vi "QCA Get Message.vi"(0 "Timeout ms (-1)":i32=-1) -> (1 "QCA Message Type":T1(ring), 2 "Text":string)   [LabVIEW 2009]
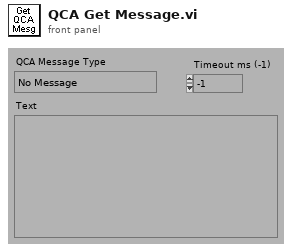
[diagram p1: front panel]
types:
  T1 = enum16{"No Message", "Bad Message", "Init", "ChannelFile=", "RF On", "RF Off", "RFFreq=", "RFMod=", "RFPower=", "YaleGain=", "ScanSweeps=", "ScanSteps=", "ScanFreq=", "CalConst=", "MonitorDelay=", "Baseline=", "Baseline", "SaveChans", "Channel=", "Pause", "TakeData", "OnePoint", "NMRTune", "Monitor", "Address=", "Ping=", "Stop"}
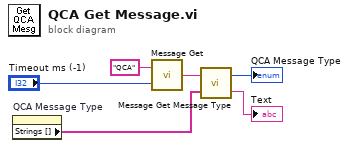
[diagram p0: block diagram]
diagram:
  n1 = property on="QCA Message Type" class="Enum (strict)"() -> ("Strings []"=w3:string[])  [unwired: 2 in, 2 out]
  n2 = call "Message Get.vi"("Timeout ms (-1)"="Timeout ms (-1)", "Module"="QCA") -> ("data out"=w6:string)
  n3 = call "Message Get Message Type.vi"("Message Types"=w3, "Message"=w6) -> ("Trailing text"=→"Text":string, "Message Type"=→"QCA Message Type":i32)
